vi "camera_pointer_mod.vi"() -> ()   [LabVIEW 2024]
uses:
  <vilib>/vision/driver/NI_Vision_Acquisition_Software.lvlib
  <resource>/objmgr/imaqdx.rc
  TCV_Lib.dll
panel:
  in  "confirm camera":bool
  out "arry_cluster":T1(array[cluster])
  out "return type":i32
  out "no_of_detections":i32
  in  "CPU:0/Gpu:1":i32=1
  in  "Class name path":path=path "C:/Users/jason/Documents/ads/tcv/TransformCV-LabVIEW/Test/model/classes.txt"
  out "Device Num":u64
  out "success_model_loading":u64
  in  "Model Path":path=path "C:/Users/jason/Documents/ads/tcv/TransformCV-LabVIEW/Test/model/nws_736_1280_b1_gpu.torchscript"
  in  "model_h":i32=736
  in  "iou":dbl=0.5
  in  "conf":dbl=0.25
  in  "frame_w":i32=1280
  in  "frame_h":i32=736
  in  "model_w":i32=1280
  out "height":u32
  out "width":u32
  out "video Mode names":string[](array[string])
  in  "Resolution Selection":u16(ring)=10 items=["640x480 MJPG 30.00fps", "640x480 YUY2 30.00fps", "1280x720 MJPG 30.00fps", "1280x720 YUY2 7.50fps", "1920x1080 MJPG 30.00fps", "1920x1080 YUY2 2.00fps", "2048x1536 MJPG 30.00fps", "2048x1536 YUY2 2.00fps", "2560x1440 MJPG 30.00fps", "2560x1440 YUY2 2.00fps", "3840x2160 MJPG 30.00fps", "3840x2160 YUY2 1.00fps"]
  in  "Camera Selection":string(combo)="cam5"
  out "Camera Index list":string[](array[string])
  out "Image Border Size":i32
  out "Pixel Size x Linewidth":i32
  out "Acquired Frames per Second":dbl
  in  "stop":bool
  out "Camera":T2(plugin-control)
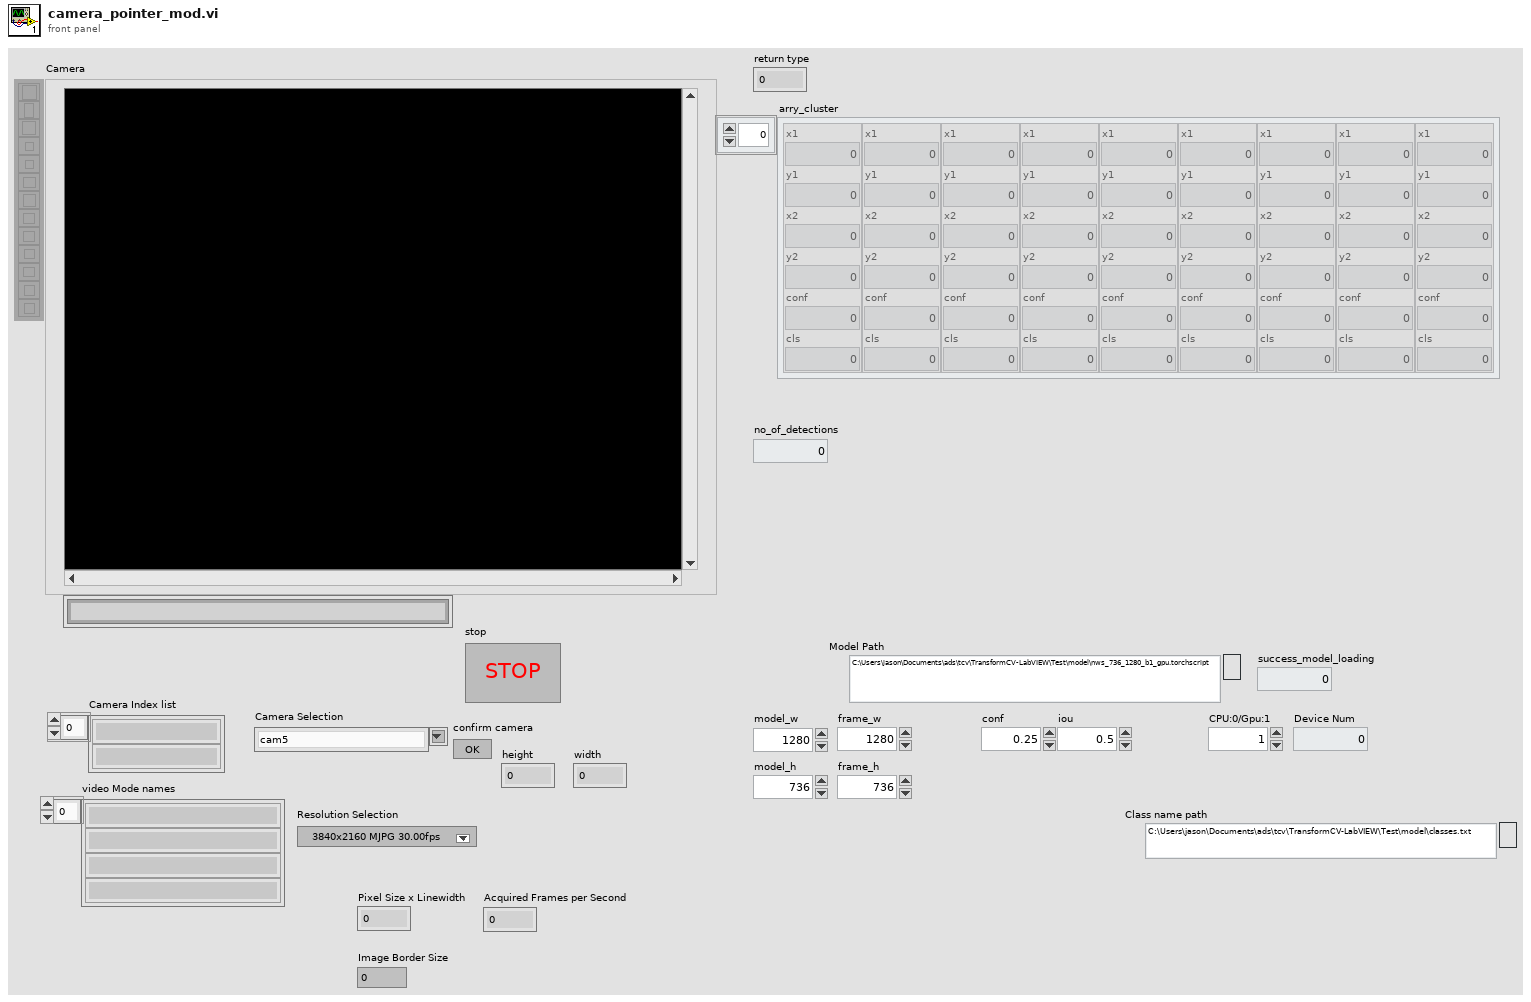
[diagram p1: front panel]
types:
  T1 = cluster{"x1":sgl, "y1":sgl, "x2":sgl, "y2":sgl, "conf":sgl, "cls":i32}[]
  T2 = typedef "IMAQ Image.ctl" = refnum<image>
  T3 = cluster{"Type":u32, "Version":u32, "Flags":u32, "SerialNumberHigh":u32, "SerialNumberLow":u32, "BusType":u32, "InterfaceName":string, "VendorName":string, "ModelName":string, "CameraFileName":string, "CameraAttributeURL":string}[]
  T4 = typedef "IMAQdx.ctl" = refnum<k21>
  T5 = cluster{"Video Mode":u32, "Video Mode Name":string}[]
  T6 = cluster{"x1":sgl, "y1":sgl, "x2":sgl, "y2":sgl, "conf":sgl, "cls":i32}
  T7 = enum32{"Map Pixel Pointer", "Unmap Pixel Pointer", "Get Pixels Infos"}
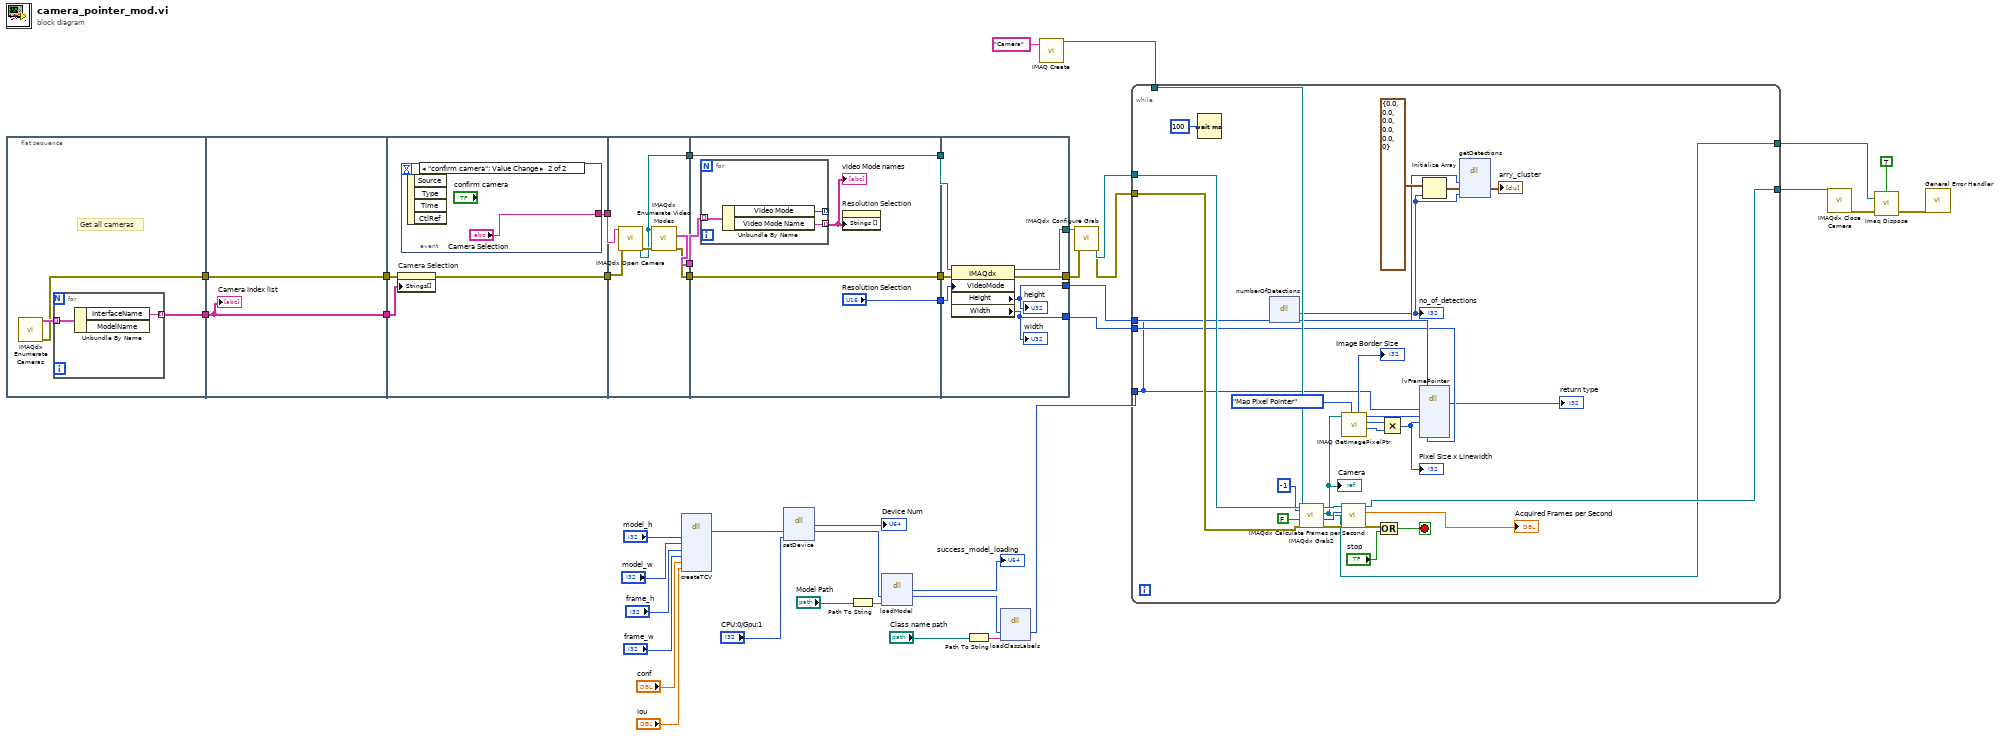
[diagram p0: block diagram]
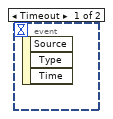
[diagram p2: hidden frame]
diagram:
  n1 = flat-sequence {
    tunnel: [w45] -> w33
    tunnel: [w43] -> w32
    tunnel: w33 -> [w49]
    tunnel: [w49] -> w31
    tunnel: [w48] -> w30
    tunnel: w32 -> [w48]
    tunnel: w31 -> [w53]
    tunnel: w30 -> [w52]
    tunnel: [w50] -> w29
    tunnel: [w51] -> w28
    tunnel: w29 -> [w60]
    tunnel: w28 -> [w59]
    tunnel: [w57] -> w27
    tunnel: [w56] -> w26
    tunnel: [w55] -> w25
    tunnel: w27 -> [w65]
    tunnel: [w63] -> w24
    tunnel: w26 -> [w63]
    tunnel: ["Resolution Selection"] -> w23
    tunnel: [w61] -> w22
    tunnel: w25 -> [w61]
    tunnel: w24 -> [w75]
    tunnel: w23 -> [w74]
    tunnel: w22 -> [w73]
    tunnel: [w72] -> w21
    tunnel: [w71] -> w20
    tunnel: [w70] -> w19
    tunnel: [w69] -> w18
    frame #0 {
      # "Get all cameras"
      n2 = call <vilib>:"IMAQdx Enumerate Cameras.vi"() -> ("error out"=w43:errorcluster, "Camera Information Array"=w44:T3)  [unwired: 10 in]
      n3 = for {
        tunnel: w44 -> [w47] mode=indexing
        tunnel: [w46] -> w45 mode=indexing
        n4 = Unbundle By Name(w47) -> ("InterfaceName"=w46:string)  [unwired: 1 out]
      }
    }
    frame #1 {
      "Camera Index list" <- w49
    }
    frame #2 {
      n5 = property on="Camera Selection" class="CmbBox"(error in=w52, "Strings[]"=w53) -> (error out=w51:errorcluster)  [unwired: 1 in, 1 out]
      n6 = event shown="[1] \"confirm camera\": Value Change" {
        selector: _ -> [_ _]
        dyn-events: _ -> [_ _]
        timeout: _ -> [_ _]
        tunnel: [_ "Camera Selection"] -> w50
        event Timeout {
          n7 = event-data() -> ()  [unwired: 1 in, 3 out]
        }
        event "confirm camera": Value Change {
          n8 = event-data() -> ()  [unwired: 1 in, 4 out]
        }
      }
    }
    frame #3 {
      n9 = call <vilib>:"IMAQdx Open Camera.vi"("error in"=w59, "Session In"=w60) -> ("error out"=w58:errorcluster, "Session Out"=w56:T4)  [unwired: 8 in]
      n10 = call <vilib>:"IMAQdx Enumerate Video Modes.vi"("error in"=w58, "Session In"=w56) -> ("error out"=w55:errorcluster, "Video Modes"=w57:T5)  [unwired: 6 in, 2 out]
    }
    frame #4 {
      n11 = for {
        tunnel: w65 -> [w68] mode=indexing
        tunnel: [w67] -> _ mode=indexing
        tunnel: [w66] -> w64 mode=indexing
        n12 = Unbundle By Name(w68) -> ("Video Mode"=w67:u32, "Video Mode Name"=w66:string)
      }
      "video Mode names" <- w64
      n13 = property on="Resolution Selection" class="Ring (strict)"("Strings []"=w64) -> ()  [unwired: 2 in, 2 out]
    }
    frame #5 {
      n14 = property class="IMAQdx"(reference=w75, error in=w73, "VideoMode"=w74) -> (reference out=w70:T4, error out=w69:errorcluster, "Height"=w71:u32, "Width"=w72:u32)
      "height" <- w71
      "width" <- w72
    }
  }
  n15 = dll-call lib="C:/Users/jason/Documents/ads/tcv/TransformCV-LabVIEW/Test/TCV_Lib.dll" fn="createTCV"("model_h"="model_h", "model_w"="model_w", "frame_h"="frame_h", "frame_w"="frame_w", "conf"="conf", "iou"="iou") -> ("return Obj"=w11:u64)  [unwired: 9 in, 2 out]
  n16 = dll-call lib="C:/Users/jason/Documents/ads/tcv/TransformCV-LabVIEW/Test/TCV_Lib.dll" fn="setDevice"("ref"=w11, "device"="CPU:0/Gpu:1") -> ("return type"=→"Device Num":u64, "ref"=w8:u64)  [unwired: 4 in, 2 out]
  n17 = Path To String(path="Model Path") -> (string=w12:string)
  n18 = dll-call lib="C:/Users/jason/Documents/ads/tcv/TransformCV-LabVIEW/Test/TCV_Lib.dll" fn="loadModel"("ref"=w8, "path"=w12) -> ("success"=→"success_model_loading":i32, "ref"=w5:u64)  [unwired: 4 in, 2 out]
  n19 = Path To String(path="Class name path") -> (string=w6:string)
  n20 = dll-call lib="C:/Users/jason/Documents/ads/tcv/TransformCV-LabVIEW/Test/TCV_Lib.dll" fn="loadClassLabels"("ref"=w5, "class_names"=w6) -> ("ref"=w1:u64)  [unwired: 5 in, 2 out]
  n21 = call "IMAQ Create"("Image Name"="Camera") -> ("New Image"=w39:T2)  [unwired: 4 in, 1 out]
  n22 = call <vilib>:"IMAQdx Configure Grab.vi"("error in"=w18, "Session In"=w19) -> ("error out"=w40:errorcluster, "Session Out"=w41:T4)  [unwired: 8 in]
  n23 = while {
    tunnel: w41 -> [w102]
    tunnel: w40 -> [w100]
    tunnel: w39 -> [w101]
    tunnel: [w93] -> w38
    tunnel: [w85] -> w37
    tunnel: w20 -> [w87]
    tunnel: w21 -> [w86]
    tunnel: w1 -> [w82]
    stop <- w105 stop-if-true
    n24 = Wait (ms)(milliseconds to wait=u32 100) -> ()  [unwired: 1 out]
    n25 = dll-call lib="C:/Users/jason/Documents/ads/tcv/TransformCV-LabVIEW/Test/TCV_Lib.dll" fn="numberOfDetections"("ref"=w82) -> ("no_of_detections"=w76:i32, "ref"=w77:u64)  [unwired: 3 in, 2 out]
    "no_of_detections" <- w76
    n26 = call <vilib>:"IMAQdx Grab2.vi"("Timeout (ms)"=-1, "error in"=w100, "Wait for Next Buffer? (Yes)"=FALSE, "Image In"=w101, "Session In"=w102) -> ("error out"=w94:errorcluster, "Buffer Number Out"=w97:u32, "Image Out"=w85:T2, "Session Out"=w98:T4)  [unwired: 3 in]
    "Camera" <- w85
    n27 = call <vilib>:"IMAQdx Calculate Frames per Second.vi"("Session In"=w98, "Buffer Number"=w97, "error in (no error)"=w94) -> ("Session Out"=w93:T4, "Acquired Frames per Second"=→"Acquired Frames per Second":dbl, "error out"=w91:errorcluster)  [unwired: 6 in, 4 out]
    n28 = call "IMAQ GetImagePixelPtr"("Function"=T7."Map Pixel Pointer", "Image"=w85) -> ("Pixel Size (Bytes)"=w84:i32, "LineWidth(Pixels)"=w90:i32, "Pixel Pointer out"=w88:u64, "Image Border Size"=→"Image Border Size":i32)  [unwired: 4 in, 2 out]
    n29 = Or(x=w91, y="stop") -> (x .or. y?=w105:bool)
    n30 = Multiply(x=w90, y=w84) -> (x*y=w83:i32)
    "Pixel Size x Linewidth" <- w83
    n31 = dll-call lib="C:/Users/jason/Documents/ads/tcv/TransformCV-LabVIEW/Test/TCV_Lib.dll" fn="lvFramePointer"("ref"=w82, "ImagePointer"=w88, "Linewidth"=w83, "h"=w87, "w"=w86) -> ("return type"=→"return type":i32)  [unwired: 8 in, 2 out]
    n32 = Initialize Array(T6 {"x1"=0.0, "y1"=0.0, "x2"=0.0, "y2"=0.0, "conf"=0.0, "cls"=0}, w76) -> (w79:T1)
    n33 = dll-call lib="C:/Users/jason/Documents/ads/tcv/TransformCV-LabVIEW/Test/TCV_Lib.dll" fn="getDetections"("ref"=w77, "arry_cluster"=w79, "numberofdetection"=w76) -> ("arry_cluster"=→"arry_cluster":T1)  [unwired: 6 in, 2 out]
  }
  n34 = call <vilib>:"IMAQdx Close Camera.vi"("Session In"=w38) -> ("error out"=w36:errorcluster)  [unwired: 10 in]
  n35 = call "Imaq Dispose"("All Images? (No)"=TRUE, "Image"=w37, "error in (no error)"=w36) -> ("error out"=w35:errorcluster)  [unwired: 3 in]
  n36 = call <vilib>:"General Error Handler.vi"("error in (no error)"=w35) -> ()  [unwired: 10 in, 5 out]
